vi "Control visibility.vi"(8 "error in (no error)":errorcluster, 10 "Setpoint type":T1, 11 "Controls[]":refnum<vi>[](array[refnum])) -> (0 "error out":errorcluster)   [LabVIEW 2020]
uses:
  Controls/Serpoint.ctl
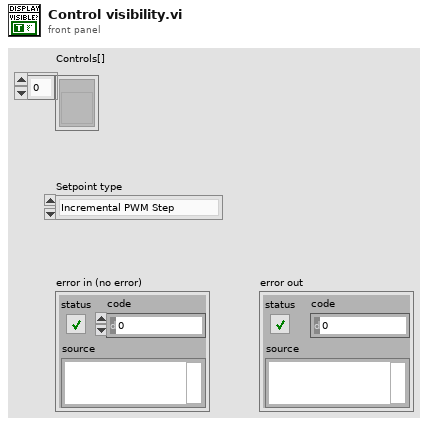
[diagram p1: front panel]
types:
  T1 = typedef "Serpoint.ctl" = enum16{"Incremental PWM Step", "PWM Step", "Ramp", "Sinusoidal", "Blood-Pressure"}
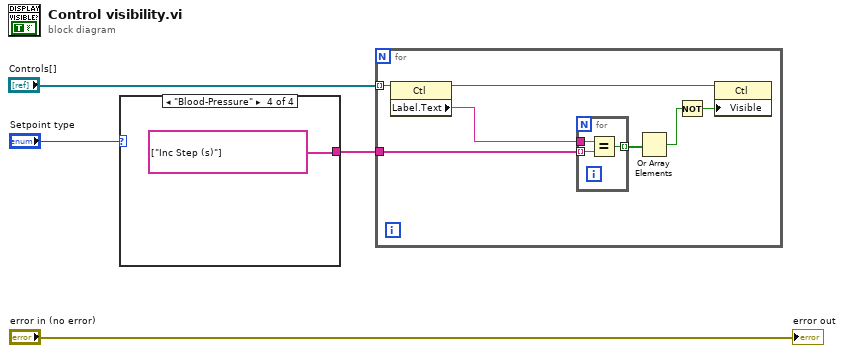
[diagram p0: block diagram]
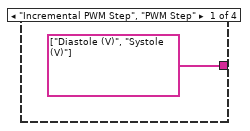
[diagram p2: hidden frame]
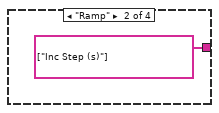
[diagram p3: hidden frame]
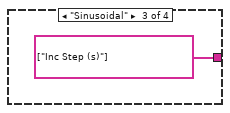
[diagram p4: hidden frame]
diagram:
  n1 = case shown="\"Blood-Pressure\"" "Setpoint type" {
    tunnel: [string[] ["Diastole (V)", "Systole (V)"] string[] ["Inc Step (s)"] string[] ["Inc Step (s)"] string[] ["Inc Step (s)"]] -> w2
    frame "Incremental PWM Step", "PWM Step" {
    }
    frame "Ramp" {
    }
    frame "Sinusoidal" {
    }
    frame "Blood-Pressure" {
    }
  }
  n2 = for {
    tunnel: w2 -> [w12]
    tunnel: "Controls[]" -> [w9] mode=indexing
    n3 = property class="Ctl"(reference=w9) -> (reference out=w10:refnum<vi>, "Label.Text"=w11:string)  [unwired: 1 in, 1 out]
    n4 = for {
      tunnel: w11 -> [w16]
      tunnel: w12 -> [w18] mode=indexing
      tunnel: [w17] -> w15 mode=indexing
      n5 = Equal?(x=w16, y=w18) -> (x = y?=w17:bool)
    }
    n6 = Or Array Elements(Boolean array=w15) -> (logical OR=w14:bool)
    n7 = Not(x=w14) -> (.not. x?=w13:bool)
    n8 = property class="Ctl"(reference=w10, "Visible"=w13) -> ()  [unwired: 1 in, 2 out]
  }
  "error out" <- "error in (no error)"
